vi "GetVersionString.vi"(3 "SetList root path":path) -> (1 "Version String":string)   [LabVIEW 2013]
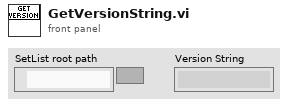
[diagram p1: front panel]
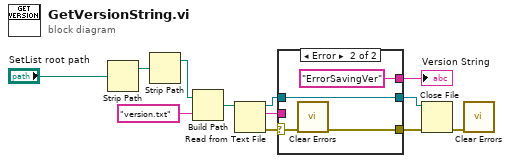
[diagram p0: block diagram]
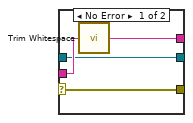
[diagram p2: hidden frame]
diagram:
  n1 = Strip Path(path="SetList root path") -> (stripped path=w8:path)  [unwired: 1 out]
  n2 = Strip Path(path=w8) -> (stripped path=w9:path)  [unwired: 1 out]
  n3 = Build Path(base path=w9, name or relative path="version.txt") -> (appended path=w11:path)
  n4 = Read from Text File(file (use dialog)=w11) -> (refnum out=w2:refnum<file>, text=w4:string, error out=w3:errorcluster)  [unwired: 3 in, 1 out]
  n5 = case shown="Error" w3 {
    selector: w3 -> [w14 w19]
    tunnel: w4 -> [w16 _]
    tunnel: [w15 "ErrorSavingVer" ("trimmed string")] -> w12
    tunnel: [w14 w18] -> w5
    tunnel: [w13 w17] -> w1
    tunnel: w2 -> [w13 w17]
    frame No Error {
      n6 = call <vilib>:"Trim Whitespace.vi"("string"=w16) -> ("trimmed string"=w15:string)  [unwired: 1 in]
    }
    frame Error {
      n7 = call <vilib>:"Clear Errors.vi"("error in (no error)"=w19) -> ("error out"=w18:errorcluster)  [unwired: 6 in]
    }
  }
  "Version String" <- w12
  n8 = Close File(refnum=w1, error in=w5) -> (error out=w6:errorcluster)  [unwired: 1 out]
  n9 = call <vilib>:"Clear Errors.vi"("error in (no error)"=w6) -> ()  [unwired: 6 in, 1 out]
